vi "680 Laser Controler and oscilloscope_v2_11.vi"() -> ()   [LabVIEW 2011]
uses:
  C:/Program Files (x86)/National Instruments/LabVIEW 2011/vi.lib/FilterByProductID/LabVIEW 2009/UsbDllWrap.dll
  Program Files (x86)/National Instruments/LabVIEW 2011/vi.lib/FilterByProductID/LabVIEW 2009/UsbDllWrap.dll
panel:
  in  "Oscilloscope read time (ms)":u32=12000
  in  "Scan time scale (s/div)":string
  in  "Reset to local scan":bool
  in  "File Type":u16(ring) items=["BIN", "TXT", "CSV"]
  in  "File Name":string
  in  "Save to File":bool
  out "Oscilloscope Error Out":errorcluster
  in  "Oscilloscope wait time (ms)":u32
  in  "laser wait time (ms)":u32=4400
  in  "Oscilloscope":refnum<visa-resource-name>="GPIB0::7::INSTR"
  out "bScan":bool=TRUE
  in  "Lambda Scan":bool=TRUE
  out "bTrack":bool=TRUE
  in  "Lambda Track":bool=TRUE
  out "bLasPwr":bool=TRUE
  in  "Laser Power":bool
  out "Laser Error Messages":i32(listbox)
  in  "Laser Power Mode":u16(ring) caption="Laser Power" items=["Constant Current", "Constant Power"]
  in  "Stop Wavelength (nm)":dbl=1570.0 min=1500.0 max=1590.0 format="%.2g"
  in  "Start Wavelength (nm)":dbl=1530.0 min=1500.0 max=1550.0 format="%.2g"
  in  "Rev. Velocity (nm/s)":dbl=10.0 min=0.0 max=8.0 format="%.2g"
  in  "Fwd. Velocity (nm/s)":dbl=9.0 min=0.0 max=20.0 format="%.2g"
  in  "Desired Scans":u16=1
  out "Scans Completed":dbl=1.0
  in  "Piezo Voltage_Set (%)":dbl=56.04 caption="Piezo Voltage (%)" format="%.2g"
  in  "Power_Set (mW)":dbl=24.0 caption="Power (mW)" format="%.2g"
  in  "Current_Set (mA)":dbl=190.0 caption="Current (mA)" format="%.2g"
  in  "Wavelength_Set (nm)":dbl=1530.0 caption="Wavelength (nm)" min=1520.0 max=1590.0 step=0.01 format="%.2g"
  out "Cavity Temp._Act (degC)":dbl=22.07 caption="Cavity Temp. (degC)" format="%.2g"
  out "Diode Temp._Act (degC)":dbl=22.136 caption="Diode Temp. (degC)" format="%.2g"
  out "Power_Act (mW)":dbl=25.818 caption="Power (mW)" format="%.2g"
  out "Current_Act (mA)":dbl=189.79 caption="Current (mA)" format="%.2g"
  out "Wavelength_Act (nm)":dbl=1529.998 caption="Wavelength (nm)"
  in  "Laser Controller":u16(ring) items=["6700 SN10081"]
  # "Scan Settings\nscan vel: 9nm; pts: 8 Mpts;\nOsc time: 5s."
  # "File Saving"
  # "Default:0"
  # "Laser Control"
  # "Actual Values"
  # "Default:4400"
  # "Save waveforms (window) to osilloscope:\nC:/Waveforms Data/\n<name>.<type>"
  # "Default:0.3"
  # "Return to local scan"
  # "Default:0.01/0.005\nBased on the function generator"
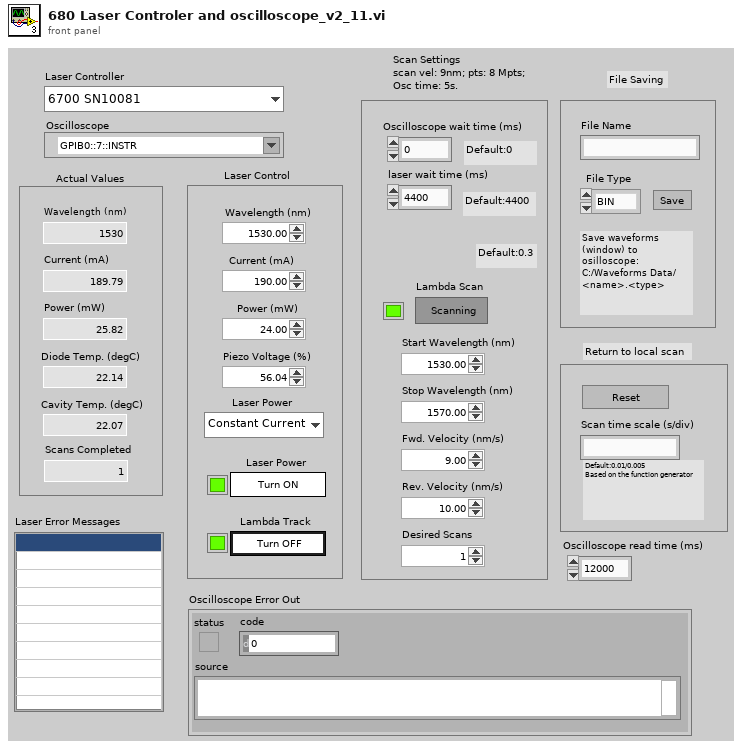
[diagram p1: front panel]
types:
  T1 = cluster{"Laser Power Mode":u16, "Start Wavelength (nm)":dbl, "Stop Wavelength (nm)":dbl, "Fwd. Velocity (nm/s)":dbl, "Rev. Velocity (nm/s)":dbl, "Desired Scans":u16, "Calibration Date:":string, "Model Number:":string, "Serial Number:":string, "Wavelength_Set (nm)":dbl, "Current_Set (mA)":dbl, "Power_Set (mW)":dbl, "Piezo Voltage_Set (%)":dbl, "Controller ID":string}
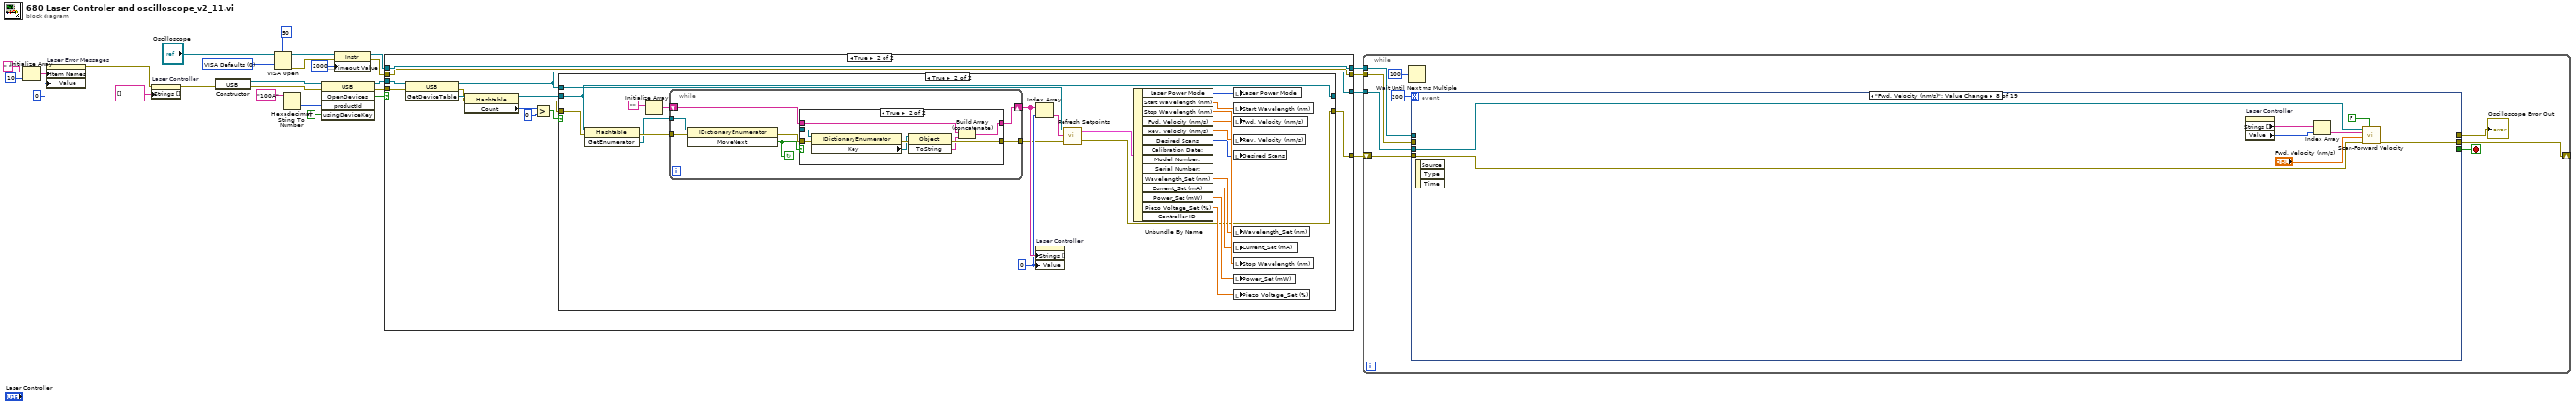
[diagram p0: block diagram]
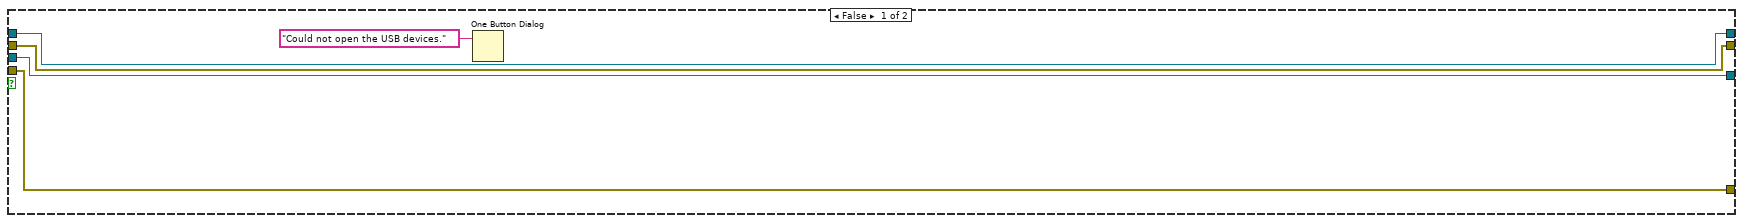
[diagram p2: hidden frame]
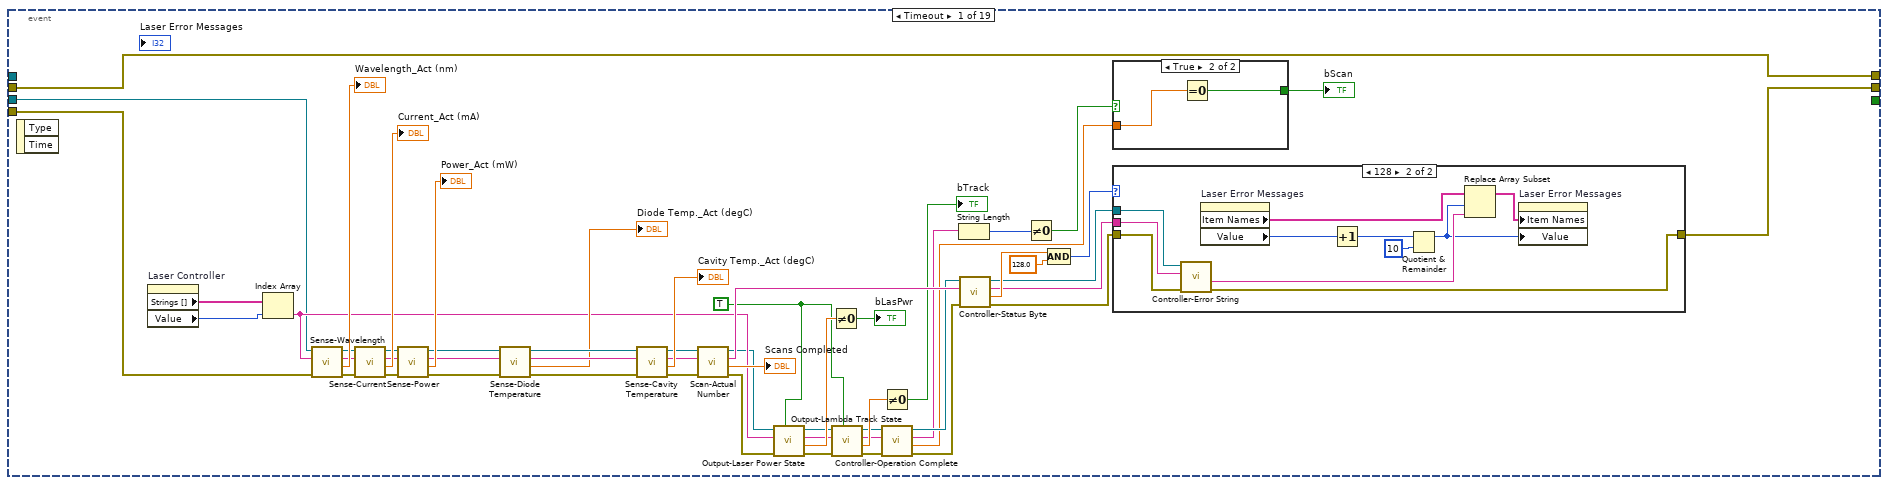
[diagram p5: hidden frame]
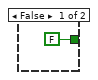
[diagram p6: hidden frame]
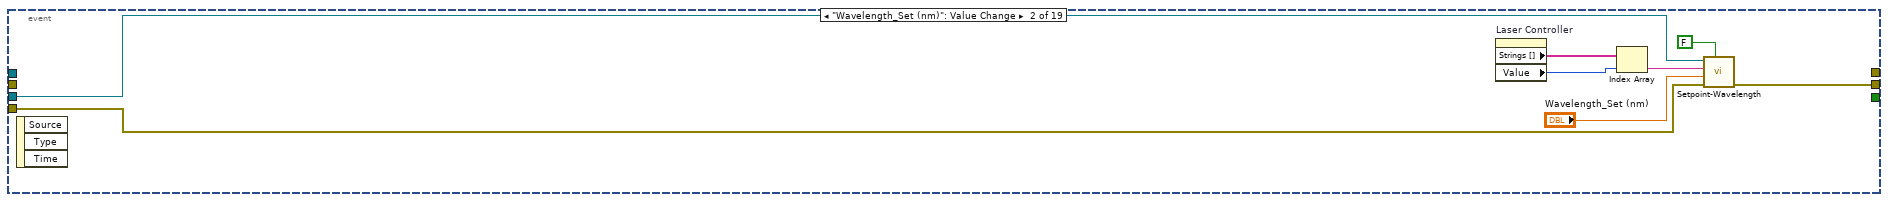
[diagram p8: hidden frame]
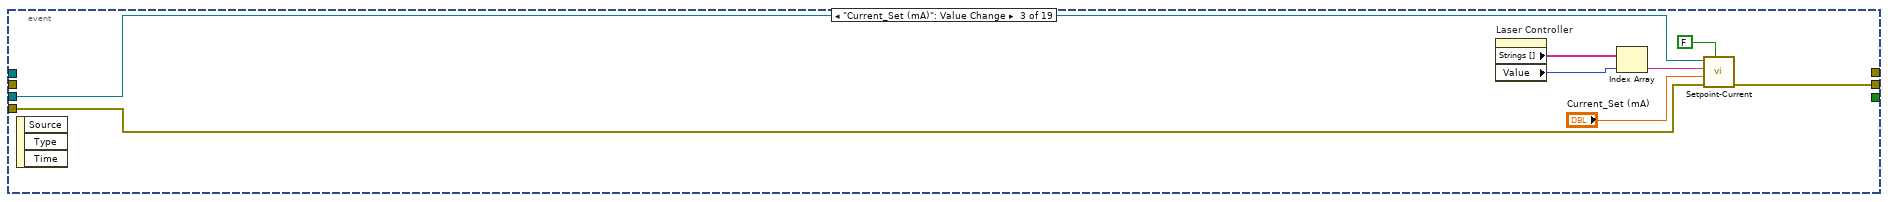
[diagram p9: hidden frame]
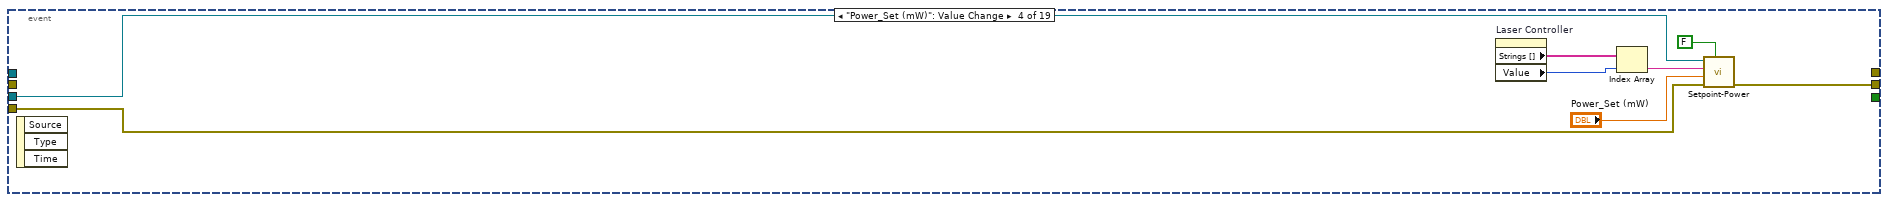
[diagram p10: hidden frame]
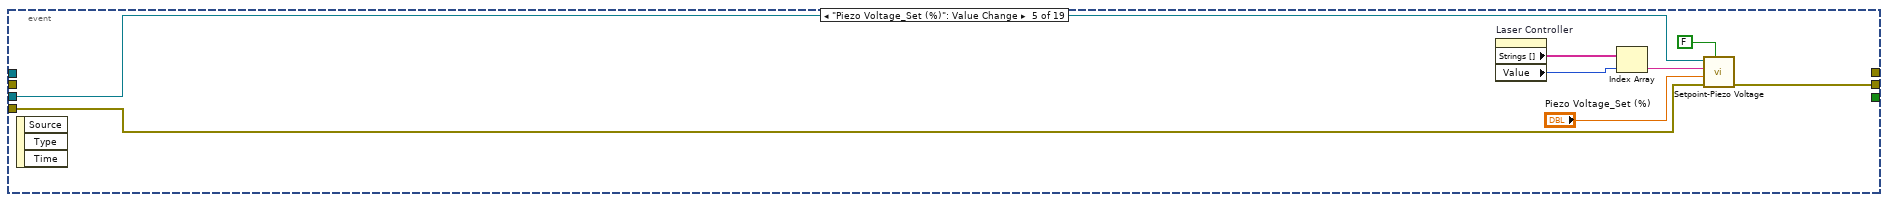
[diagram p11: hidden frame]
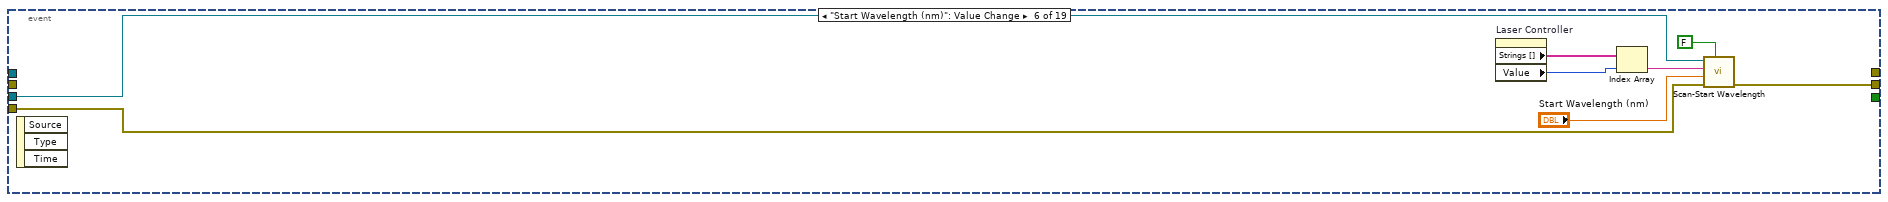
[diagram p12: hidden frame]
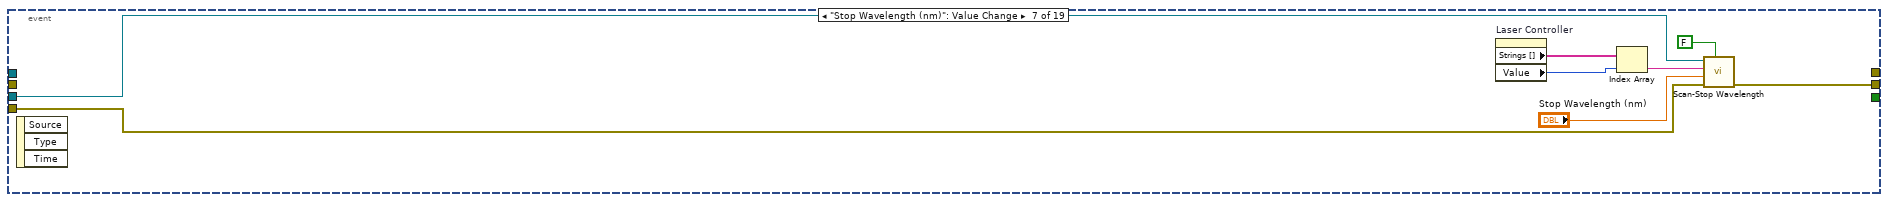
[diagram p13: hidden frame]
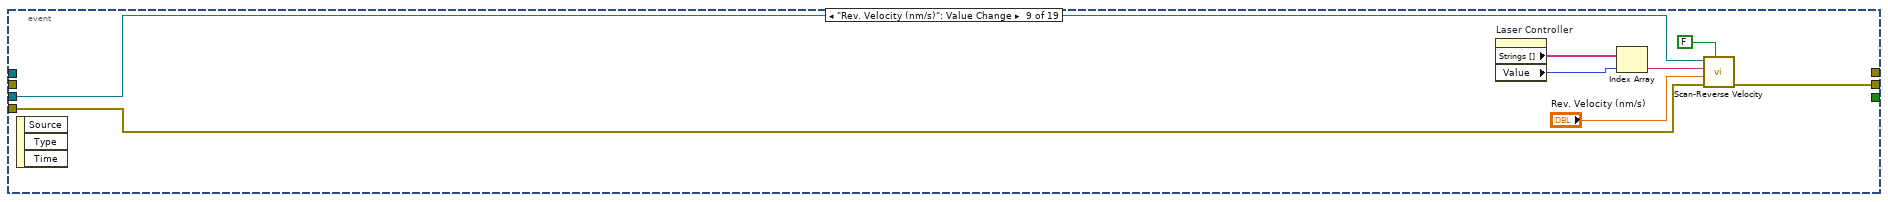
[diagram p14: hidden frame]
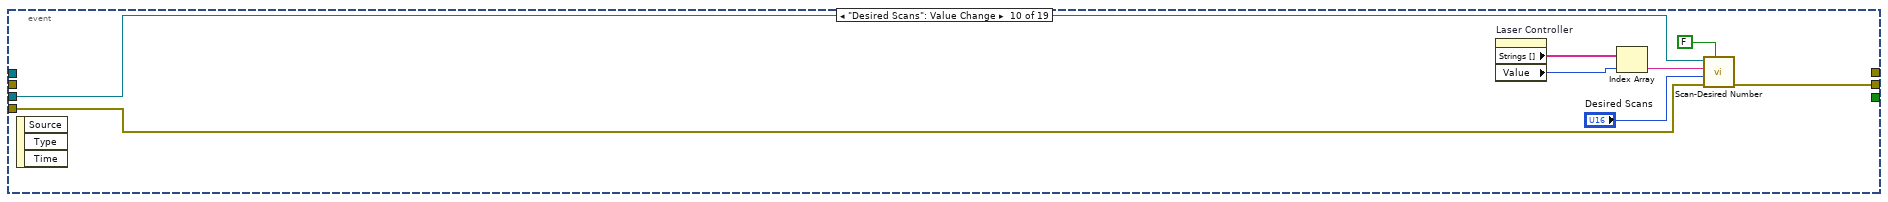
[diagram p15: hidden frame]
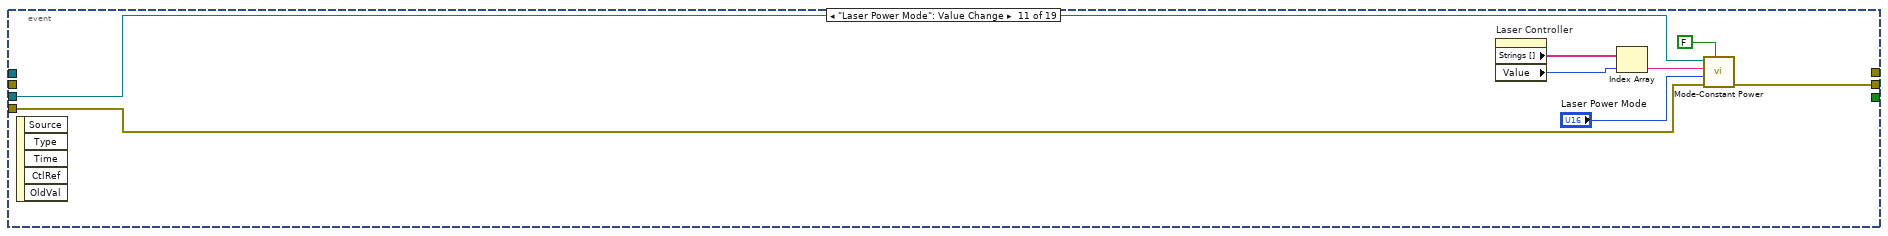
[diagram p16: hidden frame]
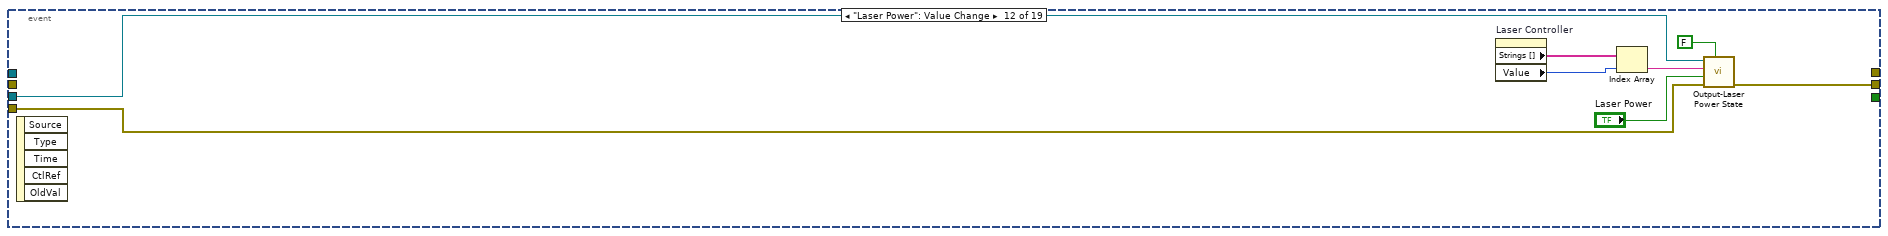
[diagram p17: hidden frame]
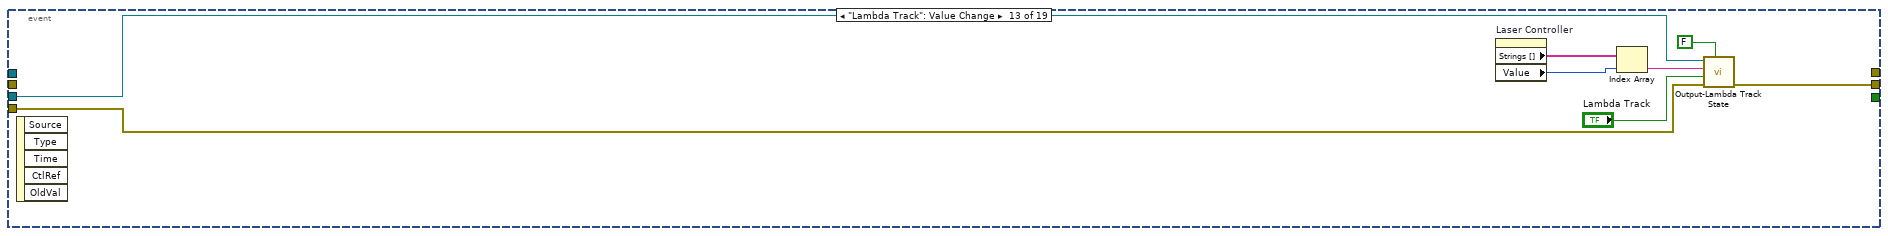
[diagram p18: hidden frame]
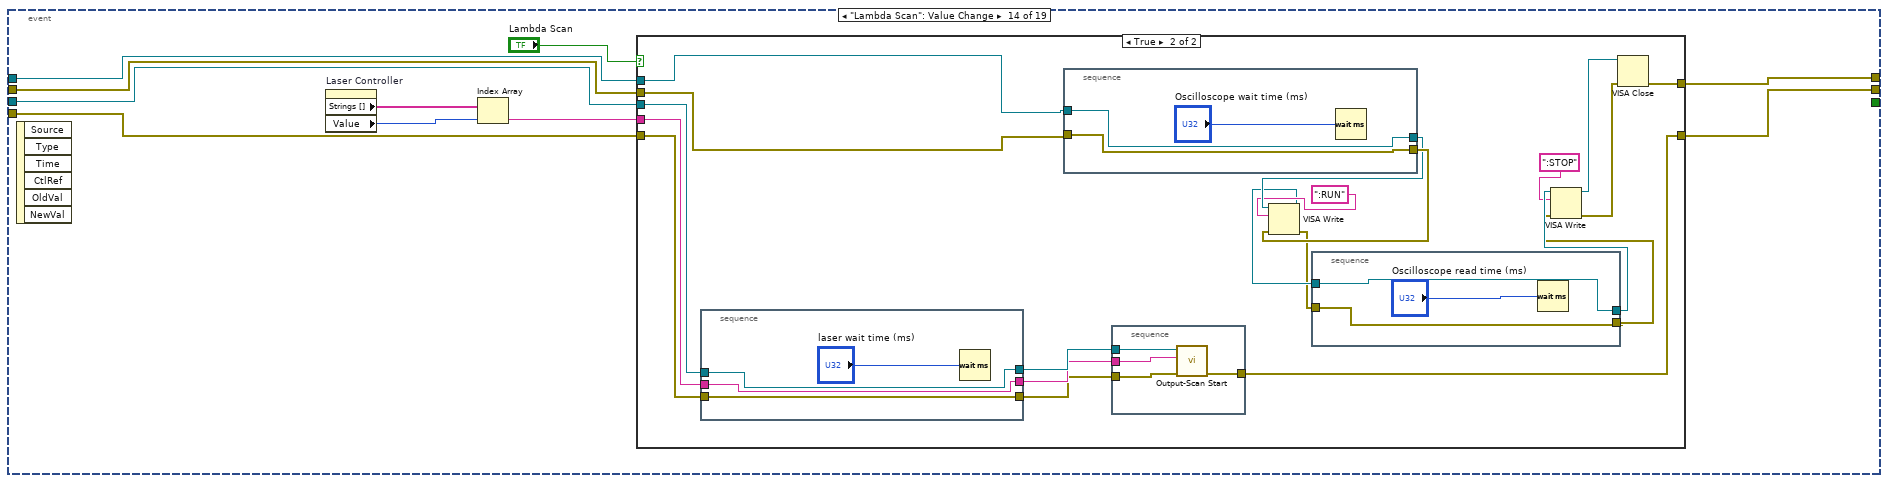
[diagram p19: hidden frame]
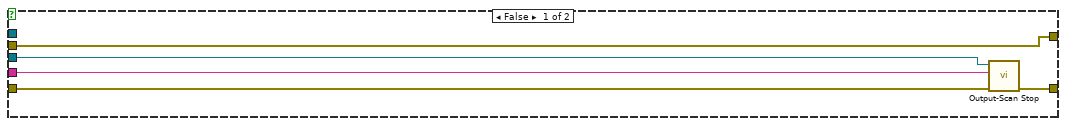
[diagram p20: hidden frame]
diagram:
  w2 = u32 0 items=["VISA Defaults"=0, "Exclusive Lock"=1, "Load Configured Settings"=4]
  n1 = Initialize Array(" ", 10 ("dimension size")) -> (w25:string[])
  n2 = property on="Laser Error Messages" class="LstBox (strict)"("Item Names"=w25, "Value"=0 ("Error Messages")) -> (error out=w23:errorcluster)  [unwired: 2 in, 1 out]
  n3 = property on="Laser Controller" class="Ring (strict)"(error in=w23, "Strings []"=string[] []) -> (error out=w13:errorcluster)  [unwired: 1 in, 1 out]
  n4 = constructor class="USB" ("Constructor Node")(error in=w13) -> (reference out=w19:refnum<k24>, error out=w18:errorcluster)  [unwired: 2 in, 1 out]
  n5 = VISA Open(timeout (0)=50, access mode=w2, VISA resource name="Oscilloscope") -> (VISA resource name=w8:refnum<visa-resource-name>, error out=w9:errorcluster)  [unwired: 2 in]
  n6 = Hexadecimal String To Number(string="100A") -> (number=w21:u32)  [unwired: 2 in, 1 out]
  n7 = invoke class="USB" method="OpenDevices"(reference=w19, error in=w18, "productId"=w21, "usingDeviceKey"=TRUE) -> (reference out=w14:refnum<k24>, error out=w15:errorcluster, "OpenDevices"=w16:bool)  [unwired: 1 in, 2 out]
  n8 = property class="Instr"(reference=w8, error in=w9, "General Settings:Timeout Value"=2000) -> (reference out=w6:refnum<visa-resource-name>, error out=w5:errorcluster)
  n9 = case shown="True" w16 {
    tunnel: w14 -> [w30 w45]
    tunnel: w15 -> [w31 w37]
    tunnel: [w31 w36] -> w11
    tunnel: [w30 w35] -> w12
    tunnel: [w28 w33] -> w10
    tunnel: [w29 w34] -> w4
    tunnel: w6 -> [w29 w34]
    tunnel: w5 -> [w28 w33]
    frame False {
      n10 = One Button Dialog(message="Could not open the USB devices.") -> ()  [unwired: 1 in, 1 out]
    }
    frame True {
      n11 = invoke class="USB" method="GetDeviceTable"(reference=w45, error in=w37) -> (reference out=w35:refnum<k24>, error out=w43:errorcluster, "GetDeviceTable"=w44:refnum<k24>)  [unwired: 1 in]
      n12 = property class="Hashtable"(reference=w44, error in=w43) -> (reference out=w39:refnum<k24>, error out=w38:errorcluster, "Count"=w41:i32)
      n13 = Greater?(x=w41, y=0) -> (0:w40:bool)
      n14 = case shown="True" w40 {
        tunnel: w38 -> [w47 w70]
        tunnel: w39 -> [w46 w65]
        tunnel: [w47 w48] -> w36
        tunnel: [w46 w65] -> _
        tunnel: w35 -> [_ w61]
        frame False {
        }
        frame True {
          w63 = 0
          n15 = invoke class="Hashtable" method="GetEnumerator"(reference=w65, error in=w70) -> (error out=w69:errorcluster, "GetEnumerator"=w68:refnum<k24>)  [unwired: 1 in, 1 out]
          n16 = Initialize Array("") -> (w66:string[])  [unwired: 1 in]
          n17 = while {
            tunnel: w69 -> [w78]
            tunnel: w68 -> [w77]
            tunnel: [w73] -> w49
            shift-right: [w71] -> w64
            shift-left: w66 -> [w72]
            stop <- w74 continue-if-true
            n18 = invoke class="IDictionaryEnumerator" method="MoveNext"(reference=w77, error in=w78) -> (reference out=w76:refnum<k24>, error out=w75:errorcluster, "MoveNext"=w74:bool)  [unwired: 1 in]
            n19 = case shown="True" w74 {
              tunnel: w76 -> [_ w88]
              tunnel: w75 -> [w80 w87]
              tunnel: [w80 w84] -> w73
              tunnel: w72 -> [w79 w83]
              tunnel: [w79 w81] -> w71
              frame False {
              }
              frame True {
                n20 = property class="IDictionaryEnumerator"(reference=w88, error in=w87) -> (error out=w86:errorcluster, "Key"=w85:refnum<k24>)  [unwired: 1 out]
                n21 = invoke class="Object" method="ToString"(reference=w85, error in=w86) -> (error out=w84:errorcluster, "ToString"=w82:string)  [unwired: 1 in, 1 out]
                n22 = Build Array (concatenate) "Build Array"(w83, w82) -> (w81:string[])
              }
            }
          }
          n23 = Index Array(array=w64, index=w63) -> (element=w62:string)
          n24 = property on="Laser Controller" class="Ring (strict)"("Strings []"=w64, "Value"=w63) -> ()  [unwired: 2 in, 2 out]
          n25 = call <vilib>:"Refresh Setpoints.vi"("error in"=w49, "DeviceKey in"=w62, "USBDLLWrap Ref In"=w61) -> ("error out"=w48:errorcluster, "Cluster"=w60:T1)
          n26 = Unbundle By Name(w60) -> ("Laser Power Mode"=w59:u16, "Start Wavelength (nm)"=w58:dbl, "Stop Wavelength (nm)"=w57:dbl, "Fwd. Velocity (nm/s)"=w56:dbl, "Rev. Velocity (nm/s)"=w55:dbl, "Desired Scans"=w54:u16, "Wavelength_Set (nm)"=w53:dbl, "Current_Set (mA)"=w52:dbl, "Power_Set (mW)"=w51:dbl, "Piezo Voltage_Set (%)"=w50:dbl)  [unwired: 4 out]
          n27 = local write "Laser Power Mode"(w59) -> ()
          n28 = local write "Start Wavelength (nm)"(w58) -> ()
          n29 = local write "Fwd. Velocity (nm/s)"(w56) -> ()
          n30 = local write "Rev. Velocity (nm/s)"(w55) -> ()
          n31 = local write "Desired Scans"(w54) -> ()
          n32 = local write "Wavelength_Set (nm)"(w53) -> ()
          n33 = local write "Current_Set (mA)"(w52) -> ()
          n34 = local write "Stop Wavelength (nm)"(w57) -> ()
          n35 = local write "Power_Set (mW)"(w51) -> ()
          n36 = local write "Piezo Voltage_Set (%)"(w50) -> ()
        }
      }
    }
  }
  n37 = while {
    shift-right: [w93] -> _
    shift-left: w11 -> [w94]
    tunnel: w12 -> [w92]
    tunnel: w10 -> [w91]
    tunnel: w4 -> [w90]
    stop <- w97 stop-if-true
    n38 = Wait Until Next ms Multiple(millisecond multiple=u32 100) -> ()  [unwired: 1 out]
    n39 = event shown="[7] \"Fwd. Velocity (nm/s)\": Value Change" {
      selector: _ -> [_ _ _ _ _ _ _ _ _ _ _ _ _ _ _ _ _ _ _]
      dyn-events: _ -> [_ _ _ _ _ _ _ _ _ _ _ _ _ _ _ _ _ _ _]
      timeout: 200 -> [_ _ _ _ _ _ _ _ _ _ _ _ _ _ _ _ _ _ _]
      tunnel: [_ _ _ _ _ _ _ _ _ _ _ _ _ _ _ _ TRUE TRUE _] -> w97
      tunnel: w94 -> [w133 w173 w181 w189 w197 w205 w213 w221 w229 w237 w245 w253 w261 w271 _ _ w346 w348 w351]
      tunnel: [w121 w170 w178 w186 w194 w202 w210 w218 w226 w234 w242 w250 w258 w270 _ _ w346 w348 w350] -> w93
      tunnel: w92 -> [w106 w168 w176 w184 w192 w200 w208 w216 w224 w232 w240 w248 w256 w269 _ _ _ _ w352]
      tunnel: w90 -> [_ _ _ _ _ _ _ _ _ _ _ _ _ w267 w320 w326 _ _ _]
      tunnel: w91 -> [w98 _ _ _ _ _ _ _ _ _ _ _ _ w266 w319 w325 _ _ _]
      tunnel: [w98 _ _ _ _ _ _ _ _ _ _ _ _ w264 w318 w324 _ _ _] -> w89
      event Timeout {
        w116 = TRUE ("Query?")
        n40 = event-data() -> ()  [unwired: 3 out]
        n41 = property on="Laser Controller" class="Ring (strict)"() -> ("Strings []"=w152:string[], "Value"=w151:u16)  [unwired: 2 in, 2 out]
        n42 = Index Array(array=w152, index=w151) -> (element=w120:string)
        n43 = call <vilib>:"Sense-Wavelength.vi"("error in"=w133, "DeviceKey in"=w120, "USBDLLWrap Ref In"=w106) -> ("error out"=w144:errorcluster, "Response"=→"Wavelength_Act (nm)":dbl, "DeviceKey out"=w148:string, "USBDLLWrap Ref Out"=w149:refnum<k24>)  [unwired: 2 out]
        n44 = call <vilib>:"Sense-Current.vi"("error in"=w144, "DeviceKey in"=w148, "USBDLLWrap Ref In"=w149) -> ("error out"=w143:errorcluster, "Response"=→"Current_Act (mA)":dbl, "DeviceKey out"=w145:string, "USBDLLWrap Ref Out"=w146:refnum<k24>)  [unwired: 2 out]
        n45 = call <vilib>:"Sense-Power.vi"("error in"=w143, "DeviceKey in"=w145, "USBDLLWrap Ref In"=w146) -> ("error out"=w141:errorcluster, "Response"=→"Power_Act (mW)":dbl, "DeviceKey out"=w140:string, "USBDLLWrap Ref Out"=w139:refnum<k24>)  [unwired: 2 out]
        n46 = call <vilib>:"Sense-Diode Temperature.vi"("error in"=w141, "DeviceKey in"=w140, "USBDLLWrap Ref In"=w139) -> ("error out"=w136:errorcluster, "Response"=→"Diode Temp._Act (degC)":dbl, "DeviceKey out"=w137:string, "USBDLLWrap Ref Out"=w138:refnum<k24>)  [unwired: 2 out]
        n47 = call <vilib>:"Sense-Cavity Temperature.vi"("error in"=w136, "DeviceKey in"=w137, "USBDLLWrap Ref In"=w138) -> ("error out"=w130:errorcluster, "Response"=→"Cavity Temp._Act (degC)":dbl, "DeviceKey out"=w131:string, "USBDLLWrap Ref Out"=w132:refnum<k24>)  [unwired: 2 out]
        n48 = call <vilib>:"Scan-Actual Number.vi"("error in"=w130, "DeviceKey in"=w131, "USBDLLWrap Ref In"=w132) -> ("error out"=w118:errorcluster, "Response"=→"Scans Completed":dbl, "DeviceKey out"=w128:string, "USBDLLWrap Ref Out"=w105:refnum<k24>)  [unwired: 2 out]
        n49 = call <vilib>:"Output-Laser Power State.vi"("Query?"=w116, "error in"=w118, "DeviceKey in"=w120, "USBDLLWrap Ref In"=w105) -> ("error out"=w112:errorcluster, "Response"=w119:dbl, "DeviceKey out"=w115:string, "USBDLLWrap Ref Out"=w117:refnum<k24>)  [unwired: 1 in]
        n50 = Not Equal To 0?(x=w119) -> (x != 0?=→"bLasPwr":bool)
        n51 = call <vilib>:"Output-Lambda Track State.vi"("Query?"=w116, "error in"=w112, "DeviceKey in"=w115, "USBDLLWrap Ref In"=w117) -> ("error out"=w108:errorcluster, "Response"=w114:dbl, "DeviceKey out"=w109:string, "USBDLLWrap Ref Out"=w110:refnum<k24>)  [unwired: 1 in]
        n52 = Not Equal To 0?(x=w114) -> (x != 0?=→"bTrack":bool)
        n53 = call <vilib>:"Controller-Operation Complete.vi"("error in"=w108, "DeviceKey in"=w109, "USBDLLWrap Ref In"=w110) -> ("error out"=w107:errorcluster, "Response"=w100:dbl, "DeviceKey out"=w103:string, "USBDLLWrap Ref Out"=w104:refnum<k24>)  [unwired: 2 out]
        n54 = String Length(string=w103) -> (length=w102:i32)
        n55 = call <vilib>:"Controller-Status Byte.vi"("error in"=w107, "DeviceKey in"=w128, "USBDLLWrap Ref In"=w104) -> ("error out"=w122:errorcluster, "Response"=w127:dbl, "DeviceKey out"=w123:string, "USBDLLWrap Ref Out"=w124:refnum<k24>)  [unwired: 2 out]
        n56 = Not Equal To 0?(x=w102) -> (x != 0?=w101:bool)
        n57 = Compound Arithmetic op=AND(w127, 128.0 ("value")) -> (w125:i32)
        n58 = case shown="True" w101 {
          tunnel: w100 -> [_ w155]
          tunnel: [FALSE w154] -> w99
          frame False {
          }
          frame True {
            n59 = Equal To 0?(x=w155) -> (x = 0?=w154:bool)
          }
        }
        "bScan" <- w99
        n60 = case shown="128" w125 {
          tunnel: w124 -> [_ w167]
          tunnel: w123 -> [_ w166]
          tunnel: w122 -> [w156 w165]
          tunnel: [w156 w162] -> w121
          frame 0, Default {
          }
          frame 128 {
            n61 = call <vilib>:"Controller-Error String.vi"("error in"=w165, "DeviceKey in"=w166, "USBDLLWrap Ref In"=w167) -> ("error out"=w162:errorcluster, "Response"=w161:string)  [unwired: 4 out]
            n62 = property on="Laser Error Messages" class="LstBox (strict)"() -> ("Item Names"=w159:string[], "Value"=w158:i32)  [unwired: 2 in, 2 out]
            n63 = Increment(x=w158) -> (x+1=w164:i32)
            n64 = Quotient & Remainder(x=w164, y=10) -> (x-y*floor(x/y)=w157:i32)  [unwired: 1 out]
            n65 = Replace Array Subset(array=w159, new element=w161, index=w157) -> (w160:string[])
            n66 = property on="Laser Error Messages" class="LstBox (strict)"("Item Names"=w160, "Value"=w157) -> ()  [unwired: 2 in, 2 out]
          }
        }
      }
      event "Wavelength_Set (nm)": Value Change {
        n67 = event-data() -> ()  [unwired: 4 out]
        n68 = property on="Laser Controller" class="Ring (strict)"() -> ("Strings []"=w175:string[], "Value"=w174:u16)  [unwired: 2 in, 2 out]
        n69 = Index Array(array=w175, index=w174) -> (element=w171:string)
        n70 = call <vilib>:"Setpoint-Wavelength.vi"("Query?"=FALSE, "error in"=w173, "Wavelength (nm)"="Wavelength_Set (nm)", "DeviceKey in"=w171, "USBDLLWrap Ref In"=w168) -> ("error out"=w170:errorcluster)  [unwired: 3 out]
      }
      event "Current_Set (mA)": Value Change {
        n71 = event-data() -> ()  [unwired: 4 out]
        n72 = property on="Laser Controller" class="Ring (strict)"() -> ("Strings []"=w183:string[], "Value"=w182:u16)  [unwired: 2 in, 2 out]
        n73 = Index Array(array=w183, index=w182) -> (element=w179:string)
        n74 = call <vilib>:"Setpoint-Current.vi"("Query?"=FALSE, "error in"=w181, "Current (mA)"="Current_Set (mA)", "DeviceKey in"=w179, "USBDLLWrap Ref In"=w176) -> ("error out"=w178:errorcluster)  [unwired: 3 out]
      }
      event "Power_Set (mW)": Value Change {
        n75 = event-data() -> ()  [unwired: 4 out]
        n76 = property on="Laser Controller" class="Ring (strict)"() -> ("Strings []"=w191:string[], "Value"=w190:u16)  [unwired: 2 in, 2 out]
        n77 = Index Array(array=w191, index=w190) -> (element=w187:string)
        n78 = call <vilib>:"Setpoint-Power.vi"("Query?"=FALSE, "error in"=w189, "Power (mW)"="Power_Set (mW)", "DeviceKey in"=w187, "USBDLLWrap Ref In"=w184) -> ("error out"=w186:errorcluster)  [unwired: 3 out]
      }
      event "Piezo Voltage_Set (%)": Value Change {
        n79 = event-data() -> ()  [unwired: 4 out]
        n80 = property on="Laser Controller" class="Ring (strict)"() -> ("Strings []"=w199:string[], "Value"=w198:u16)  [unwired: 2 in, 2 out]
        n81 = Index Array(array=w199, index=w198) -> (element=w195:string)
        n82 = call <vilib>:"Setpoint-Piezo Voltage.vi"("Query?"=FALSE, "error in"=w197, "Piezo Voltage (%)"="Piezo Voltage_Set (%)", "DeviceKey in"=w195, "USBDLLWrap Ref In"=w192) -> ("error out"=w194:errorcluster)  [unwired: 3 out]
      }
      event "Start Wavelength (nm)": Value Change {
        n83 = event-data() -> ()  [unwired: 4 out]
        n84 = property on="Laser Controller" class="Ring (strict)"() -> ("Strings []"=w207:string[], "Value"=w206:u16)  [unwired: 2 in, 2 out]
        n85 = Index Array(array=w207, index=w206) -> (element=w203:string)
        n86 = call <vilib>:"Scan-Start Wavelength.vi"("Query?"=FALSE, "error in"=w205, "Scan Start Wavelength (nm)"="Start Wavelength (nm)", "DeviceKey in"=w203, "USBDLLWrap Ref In"=w200) -> ("error out"=w202:errorcluster)  [unwired: 3 out]
      }
      event "Stop Wavelength (nm)": Value Change {
        n87 = event-data() -> ()  [unwired: 4 out]
        n88 = property on="Laser Controller" class="Ring (strict)"() -> ("Strings []"=w215:string[], "Value"=w214:u16)  [unwired: 2 in, 2 out]
        n89 = Index Array(array=w215, index=w214) -> (element=w211:string)
        n90 = call <vilib>:"Scan-Stop Wavelength.vi"("Query?"=FALSE, "error in"=w213, "Scan Stop Wavelength (nm)"="Stop Wavelength (nm)", "DeviceKey in"=w211, "USBDLLWrap Ref In"=w208) -> ("error out"=w210:errorcluster)  [unwired: 3 out]
      }
      event "Fwd. Velocity (nm/s)": Value Change {
        n91 = event-data() -> ()  [unwired: 4 out]
        n92 = property on="Laser Controller" class="Ring (strict)"() -> ("Strings []"=w223:string[], "Value"=w222:u16)  [unwired: 2 in, 2 out]
        n93 = Index Array(array=w223, index=w222) -> (element=w219:string)
        n94 = call <vilib>:"Scan-Forward Velocity.vi"("Query?"=FALSE, "error in"=w221, "Scan Fwd. Vel. (nm/s)"="Fwd. Velocity (nm/s)", "DeviceKey in"=w219, "USBDLLWrap Ref In"=w216) -> ("error out"=w218:errorcluster)  [unwired: 3 out]
      }
      event "Rev. Velocity (nm/s)": Value Change {
        n95 = event-data() -> ()  [unwired: 4 out]
        n96 = property on="Laser Controller" class="Ring (strict)"() -> ("Strings []"=w231:string[], "Value"=w230:u16)  [unwired: 2 in, 2 out]
        n97 = Index Array(array=w231, index=w230) -> (element=w227:string)
        n98 = call <vilib>:"Scan-Reverse Velocity.vi"("Query?"=FALSE, "error in"=w229, "Scan Rev. Vel. (nm/s)"="Rev. Velocity (nm/s)", "DeviceKey in"=w227, "USBDLLWrap Ref In"=w224) -> ("error out"=w226:errorcluster)  [unwired: 3 out]
      }
      event "Desired Scans": Value Change {
        n99 = event-data() -> ()  [unwired: 4 out]
        n100 = property on="Laser Controller" class="Ring (strict)"() -> ("Strings []"=w239:string[], "Value"=w238:u16)  [unwired: 2 in, 2 out]
        n101 = Index Array(array=w239, index=w238) -> (element=w235:string)
        n102 = call <vilib>:"Scan-Desired Number.vi"("Query?"=FALSE, "error in"=w237, "Desired Number of Scans"="Desired Scans", "DeviceKey in"=w235, "USBDLLWrap Ref In"=w232) -> ("error out"=w234:errorcluster)  [unwired: 3 out]
      }
      event "Laser Power Mode": Value Change {
        n103 = event-data() -> ()  [unwired: 6 out]
        n104 = property on="Laser Controller" class="Ring (strict)"() -> ("Strings []"=w247:string[], "Value"=w246:u16)  [unwired: 2 in, 2 out]
        n105 = Index Array(array=w247, index=w246) -> (element=w243:string)
        n106 = call <vilib>:"Mode-Constant Power.vi"("Query?"=FALSE, "error in"=w245, "Mode"="Laser Power Mode", "DeviceKey in"=w243, "USBDLLWrap Ref In"=w240) -> ("error out"=w242:errorcluster)  [unwired: 3 out]
      }
      event "Laser Power": Value Change {
        n107 = event-data() -> ()  [unwired: 6 out]
        n108 = property on="Laser Controller" class="Ring (strict)"() -> ("Strings []"=w255:string[], "Value"=w254:u16)  [unwired: 2 in, 2 out]
        n109 = Index Array(array=w255, index=w254) -> (element=w251:string)
        n110 = call <vilib>:"Output-Laser Power State.vi"("Query?"=FALSE, "error in"=w253, "Laser Power State"="Laser Power", "DeviceKey in"=w251, "USBDLLWrap Ref In"=w248) -> ("error out"=w250:errorcluster)  [unwired: 3 out]
      }
      event "Lambda Track": Value Change {
        n111 = event-data() -> ()  [unwired: 6 out]
        n112 = property on="Laser Controller" class="Ring (strict)"() -> ("Strings []"=w263:string[], "Value"=w262:u16)  [unwired: 2 in, 2 out]
        n113 = Index Array(array=w263, index=w262) -> (element=w259:string)
        n114 = call <vilib>:"Output-Lambda Track State.vi"("Query?"=FALSE, "error in"=w261, "Lambda Track State"="Lambda Track", "DeviceKey in"=w259, "USBDLLWrap Ref In"=w256) -> ("error out"=w258:errorcluster)  [unwired: 3 out]
      }
      event "Lambda Scan": Value Change {
        n115 = event-data() -> ()  [unwired: 7 out]
        n116 = property on="Laser Controller" class="Ring (strict)"() -> ("Strings []"=w268:string[], "Value"=w273:u16)  [unwired: 2 in, 2 out]
        n117 = Index Array(array=w268, index=w273) -> (element=w272:string)
        n118 = case shown="True" "Lambda Scan" {
          tunnel: w269 -> [w278 w297]
          tunnel: w272 -> [w277 w295]
          tunnel: w271 -> [w276 w293]
          tunnel: [w275 w298] -> w270
          tunnel: w267 -> [_ w280]
          tunnel: w266 -> [w274 w279]
          tunnel: [w274 w291] -> w264
          frame False {
            n119 = call <vilib>:"Output-Scan Stop.vi"("error in"=w276, "DeviceKey in"=w277, "USBDLLWrap Ref In"=w278) -> ("error out"=w275:errorcluster)  [unwired: 5 out]
          }
          frame True {
            n120 = stacked-sequence {
              tunnel: [w307] -> w296
              tunnel: w297 -> [w307]
              tunnel: [w306] -> w294
              tunnel: w295 -> [w306]
              tunnel: [w305] -> w292
              tunnel: w293 -> [w305]
              frame #0 {
                n121 = Wait (ms)(milliseconds to wait="laser wait time (ms)") -> ()  [unwired: 1 out]
              }
            }
            n122 = stacked-sequence {
              tunnel: [w303] -> w289
              tunnel: w280 -> [w303]
              tunnel: [w302] -> w290
              tunnel: w279 -> [w302]
              frame #0 {
                n123 = Wait (ms)(milliseconds to wait="Oscilloscope wait time (ms)") -> ()  [unwired: 1 out]
              }
            }
            n124 = stacked-sequence {
              tunnel: [w309] -> w298
              tunnel: w296 -> [w312]
              tunnel: w294 -> [w311]
              tunnel: w292 -> [w310]
              frame #0 {
                n125 = call <vilib>:"Output-Scan Start.vi"("error in"=w310, "DeviceKey in"=w311, "USBDLLWrap Ref In"=w312) -> ("error out"=w309:errorcluster)  [unwired: 1 in, 4 out]
              }
            }
            n126 = VISA Write(VISA resource name=w289, write buffer=":RUN" ("string to write"), error in (no error)=w290) -> (VISA resource name out=w287:refnum<visa-resource-name>, error out=w286:errorcluster)  [unwired: 1 out]
            n127 = stacked-sequence {
              tunnel: [w299] -> w285
              tunnel: w287 -> [w299]
              tunnel: [w300] -> w284
              tunnel: w286 -> [w300]
              frame #0 {
                n128 = Wait (ms)(milliseconds to wait="Oscilloscope read time (ms)") -> ()  [unwired: 1 out]
              }
            }
            n129 = VISA Write(VISA resource name=w285, write buffer=":STOP", error in (no error)=w284) -> (VISA resource name out=w283:refnum<visa-resource-name>, error out=w282:errorcluster)  [unwired: 1 out]
            n130 = VISA Close(VISA resource name=w283, error in (no error)=w282) -> (error out=w291:errorcluster)
          }
        }
      }
      event "Reset to local scan": Mouse Down {
        n131 = event-data() -> ()  [unwired: 9 out]
        n132 = Concatenate Strings(":tim:pos 0;scal ", "Scan time scale (s/div)") -> (w323:string)
        n133 = VISA Write(VISA resource name=w320, write buffer=w323, error in (no error)=w319) -> (VISA resource name out=w317:refnum<visa-resource-name>, error out=w316:errorcluster)  [unwired: 1 out]
        n134 = VISA Write(VISA resource name=w317, write buffer=":run", error in (no error)=w316) -> (VISA resource name out=w314:refnum<visa-resource-name>, error out=w315:errorcluster)  [unwired: 1 out]
        n135 = VISA Close(VISA resource name=w314, error in (no error)=w315) -> (error out=w318:errorcluster)
      }
      event "Save to File": Value Change {
        n136 = event-data() -> ()  [unwired: 7 out]
        n137 = case shown="True" "Save to File" {
          tunnel: [w328 w343] -> w324
          tunnel: w326 -> [_ w331]
          tunnel: w325 -> [w328 w333]
          frame False {
          }
          frame True {
            n138 = Concatenate Strings(":DISK:SAVE:WAV ALL,\"C:/Waveforms data/", "File Name", "\",") -> (w338:string)
            n139 = Pick Line(string ("")=w338, multi-line string="BIN\nTXT\nCSV", line index="File Type") -> (output string=w337:string)
            n140 = Concatenate Strings(w337, ",ON") -> (w334:string)
            n141 = VISA Write(VISA resource name=w331, write buffer=":wav:view wind", error in (no error)=w333) -> (VISA resource name out=w330:refnum<visa-resource-name>, error out=w332:errorcluster)  [unwired: 1 out]
            n142 = VISA Write(VISA resource name=w330, write buffer=w334, error in (no error)=w332) -> (VISA resource name out=w342:refnum<visa-resource-name>, error out=w344:errorcluster)  [unwired: 1 out]
            n143 = VISA Close(VISA resource name=w342, error in (no error)=w344) -> (error out=w343:errorcluster)
          }
        }
      }
      event Application Instance Close? {
        n144 = event-data() -> ()  [unwired: 5 out]
        n145 = event-data() -> ()  [unwired: 1 in, 3 out]
      }
      event Panel Close? {
        n146 = event-data() -> ()  [unwired: 4 out]
        n147 = event-data() -> ()  [unwired: 1 in, 2 out]
      }
      event "Laser Controller": Value Change {
        n148 = event-data() -> ("NewVal"=w365:u16)  [unwired: 1 out]
        n149 = property on="Laser Controller" class="Ring (strict)"() -> ("Strings []"=w366:string[])  [unwired: 2 in, 2 out]
        n150 = Index Array(array=w366, index=w365) -> (element=w353:string)
        n151 = call <vilib>:"Refresh Setpoints.vi"("error in"=w351, "DeviceKey in"=w353, "USBDLLWrap Ref In"=w352) -> ("error out"=w350:errorcluster, "Cluster"=w364:T1)
        n152 = Unbundle By Name(w364) -> ("Laser Power Mode"=w363:u16, "Start Wavelength (nm)"=w362:dbl, "Stop Wavelength (nm)"=w361:dbl, "Fwd. Velocity (nm/s)"=w360:dbl, "Rev. Velocity (nm/s)"=w359:dbl, "Desired Scans"=w358:u16, "Wavelength_Set (nm)"=w357:dbl, "Current_Set (mA)"=w356:dbl, "Power_Set (mW)"=w355:dbl, "Piezo Voltage_Set (%)"=w354:dbl)  [unwired: 4 out]
        n153 = local write "Fwd. Velocity (nm/s)"(w360) -> ()
        n154 = local write "Rev. Velocity (nm/s)"(w359) -> ()
        n155 = local write "Desired Scans"(w358) -> ()
        n156 = local write "Wavelength_Set (nm)"(w357) -> ()
        n157 = local write "Current_Set (mA)"(w356) -> ()
        n158 = local write "Laser Power Mode"(w363) -> ()
        n159 = local write "Start Wavelength (nm)"(w362) -> ()
        n160 = local write "Stop Wavelength (nm)"(w361) -> ()
        n161 = local write "Power_Set (mW)"(w355) -> ()
        n162 = local write "Piezo Voltage_Set (%)"(w354) -> ()
      }
    }
    "Oscilloscope Error Out" <- w89
  }
